vi "Build Connection.vi"(6 "Password":string, 8 "error in (no error)":errorcluster, 9 "Username":string, 10 "*.udl file path":path, 11 "UDL Connection in":refnum<class "UDL Connection.lvclass">) -> (0 "error out":errorcluster, 3 "UDL Connection out":refnum<class "UDL Connection.lvclass">)   [LabVIEW 2020, in "ADODB.lvlib" / "UDL Connection.lvclass"]
uses:
  UDL Connection.lvclass
  UDL Connection.lvclass/UDL Connection.ctl
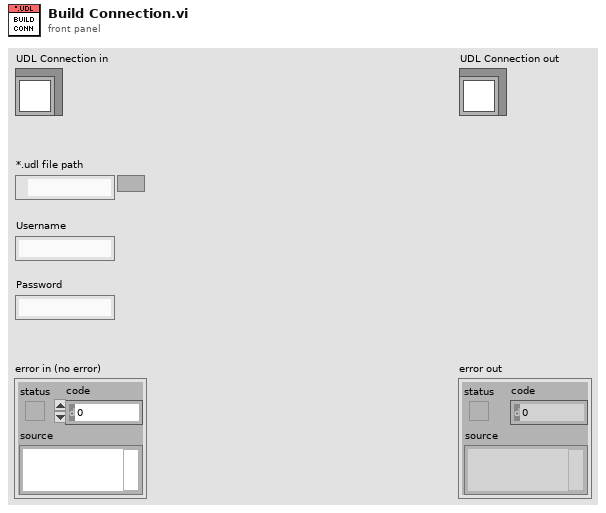
[diagram p1: front panel]
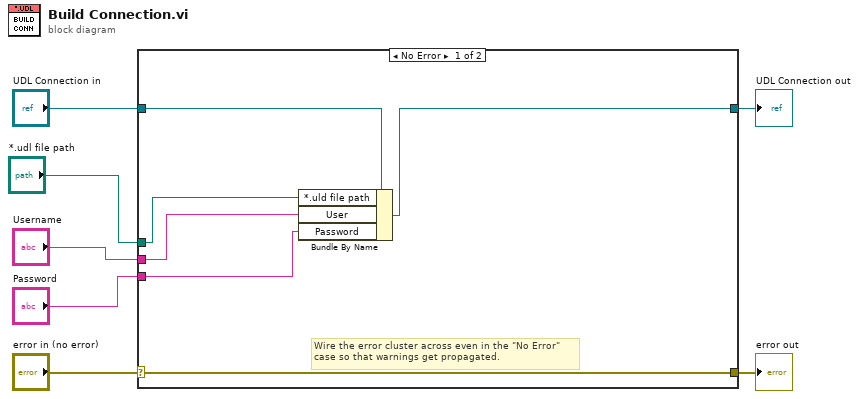
[diagram p0: block diagram]
diagram:
  n1 = case shown="No Error" "error in (no error)" {
    selector: "error in (no error)" -> [w13 w15]
    tunnel: [w13 w15] -> w6
    tunnel: [w11 w14] -> w4
    tunnel: "UDL Connection in" -> [w12 w14]
    tunnel: "*.udl file path" -> [w10 _]
    tunnel: "Username" -> [w9 _]
    tunnel: "Password" -> [w8 _]
    frame No Error {
      # "Wire the error cluster across even in the \"No Error\"\ncase so that warnings get propagated."
      n2 = Bundle By Name(cluster=w12, "*.uld file path"=w10, "User"=w9, "Password"=w8) -> (w11:refnum<class "UDL Connection.lvclass">)
    }
    frame Error {
    }
  }
  "error out" <- w6
  "UDL Connection out" <- w4
